vi "TSL_Sample.vi"() -> ()   [LabVIEW 2017]
uses:
  C:/Users/Ssantec_Test/Documents/Instrument_DLL_Sample_Labview_20250826_Ver1.5.0_x64/DLL/InstrumentDLL.dll
  DLL/InstrumentDLL.dll
  <vilib>/Utility/miscctls.llb/LVStringsAndValuesArrayTypeDef_DBL.ctl
  <vilib>/Utility/file.llb/Write To Spreadsheet File (DBL).vi
panel:
  in  "选项卡控件":T1(tab)
  in  "btnUsb_resouce":bool
  out "USB device number":string
  in  "Usb resouce":u16(ring)
  out "SweepSpeed Range":string
  in  "Port number":dbl
  in  "Target":enum32{"rdo550", "rdo570", "rdo770"}(radio)
  in  "btnSplit":bool
  out "GPIB Address":dbl
  out "GPIB Board":dbl
  in  "btnGet_Visa":bool
  in  "Visa String":u16(ring)
  in  "Communication":T2(radio)
  in  "Terminator":enum32{"rdiCr", "rdiLf", "rdiCrLf"}(radio)
  out "Serial":string
  out "Product":string
  out "F/ W Vesion":string
  out "Frequency range":string
  out "Wavelength range":string
  out "APC Limit(dBm)":string
  out "APC Limit(mW)":string
  out "ATT range":string
  in  "Btn_Connect":bool
  in  "Btn_DisConnect":bool
  in  "Address/Device number":string
  out "unit":enum16{"dBm", "mW", ""}(ring)=enum.""
  out "txtshutter":enum16{"Shutter_Open", "Shutter_Close", ""}(ring)=enum.""
  out "status":enum16{"Coh_OFF", "Coh_ON", ""}(ring)=enum.""
  out "mode":enum16{"ACC", "APC", ""}(ring)=enum.""
  out "txtlds":enum16{"LD_OFF", "LD_ON", ""}(ring)=enum.""
  out "LAN Port number":i32
  in  "Get LAN Port":bool
  out "IP Address":string
  in  "Get IP Address":bool
  in  "BtnLD_ON":bool
  in  "BtnLD_OFF":bool
  in  "BtnCoh_ON":bool
  in  "BtnCoh_OFF":bool
  in  "BtnShutter_Open":bool
  in  "BtnShutter_Close":bool
  in  "BtnAPC":bool
  in  "BtnACC":bool
  in  "BtndBm":bool
  in  "BtnmW":bool
  in  "Setting ATT":dbl
  in  "Btn_SetATT":bool
  in  "Setting Power":dbl
  in  "Btn_SetdBm":bool
  in  "Btn_SetmW":bool
  in  "Btn_GetLD":bool
  in  "BtnPower_mode":bool
  in  "BtnCoh_Status":bool
  in  "BtnShutter_Status":bool
  in  "BtnUnit":bool
  out "txtreadatt":dbl
  in  "BtnAtt_value":bool
  out "txtreadpow":dbl
  in  "BtnPower_dBm":bool
  out "txtreadmw":dbl
  in  "BtnPower_mW":bool
  out "txtreadmoni":dbl
  in  "Btnmonitor_dBm":bool
  out "txtradmoni_mw":dbl
  in  "Btnmonitor_mW":bool
  in  "txtsetwave":dbl
  in  "Btn_SetWavelength":bool
  in  "txtsetfreq":dbl
  in  "Btn_SetFrequency":bool
  in  "txtsetft":dbl
  in  "Btn_SetFinetuning":bool
  in  "Btn_Wavelength":bool
  in  "Btn_Frequency":bool
  in  "Btn_Fine":bool
  out "txtwave":dbl
  out "txtfreq":dbl
  out "txtfine":dbl
  out "txtbusy":string
  in  "Btn_Busy":bool
  in  "Wait time(msec)":i32
  in  "Btn_Stangby":bool
  out "txttsl_err":string
  in  "Btn_error":bool
  out "Start mode":enum16{"Normal", "WaitingforTrigger", ""}(ring)=enum.""
  out "Trigger output":enum16{"None", "Stop", "Start", "Step", ""}(ring)=enum.""
  out "Trigger input":enum16{"Disable", "Enable", ""}(ring)=enum.""
  out "Sweep Mode":T3(ring)=enum.""
  out "txtg_sweep_su":T4(ring)=enum."Returning"
  out "Trigger Source":enum16{"Wavelength", "Time", ""}(ring)=enum.""
  in  "Speed(570)":u16(ring) caption="Speed(nm/sec)" items=["1"=1, "2"=2, "5"=5, "10"=10, "20"=20, "50"=50, "100"=100, "200"=200]
  in  "Speed":u16(ring)
  in  "Get speed table":bool
  in  "cmbTrigger_Source":u16(ring) caption="Trigger Source(570)" items=["Wavelength", "Time", ""]
  in  "txtstart":dbl caption="Start wavelength"
  in  "Btn_SetWavelength_Parameters":bool
  in  "txtstop":dbl caption="Stop wavelength"
  in  "txtstep":dbl=0.1 caption="Trigger/wave step"
  in  "txtspeed(550)":dbl caption="Speed(nm/sec)"
  in  "Btn_Other":bool
  in  "txtdelay":dbl caption="Delay time(sec)"
  in  "txtcycle":i32=1 caption="cycle"
  in  "cmbsm":u16(ring) caption="Sweep Mode" items=["Step one way", "Continuous one way", "Step round trip", "Continuous round trip"]
  in  "cmbst_mod":u16(ring) caption="Trigger input" items=["Disable", "Enable"]
  in  "cmbtout":u16(ring) caption="Trigger output" items=["None", "Stop", "Start", "Step"]
  in  "cmbtin":u16(ring) caption="Start mode" items=["Normal", "Waiting for Trigger"]
  out "Start wavelength":dbl
  out "Stop wavelength":dbl
  out "Wavelength step":dbl
  out "Trigger step":dbl
  out "Speed(nm/sec)":dbl
  out "Delay time(sec)":dbl
  out "cycle":i32
  in  "BtnGet_setting":bool
  in  "Status":u16(ring) items=["Standby", "Running", "Pauseing", "WaitingforTrigger", "Returning"]
  in  "Wait time(msec)":i32
  in  "Btn_Waiting":bool
  in  "Btn_Status":bool
  in  "Btn_Minstep":bool
  in  "txtspeed":dbl
  out "txtcurrentc":i32
  in  "Btn_Current":bool
  in  "Btn_Start":bool
  in  "Btn_Stop":bool
  in  "Btn_SoftwareTrigger":bool
  in  "Btn_Pause":bool
  in  "Btn_ReStart":bool
  in  "Btn_GetLogg":bool
  out "TSL":refnum<k24>
  # "0. Connect Tool"
  # "1. Connect"
  # "Information"
  # "Power Control"
  # "Power status"
  # "Wavelength Control"
  # "Wavelength Status"
  # "Common Function"
  # "Sweep Setting"
  # "Other"
  # "Wavelength parameters"
  # "Other parameters"
  # "Sweep Speed(nm/s)"
  # "Sweep setting status"
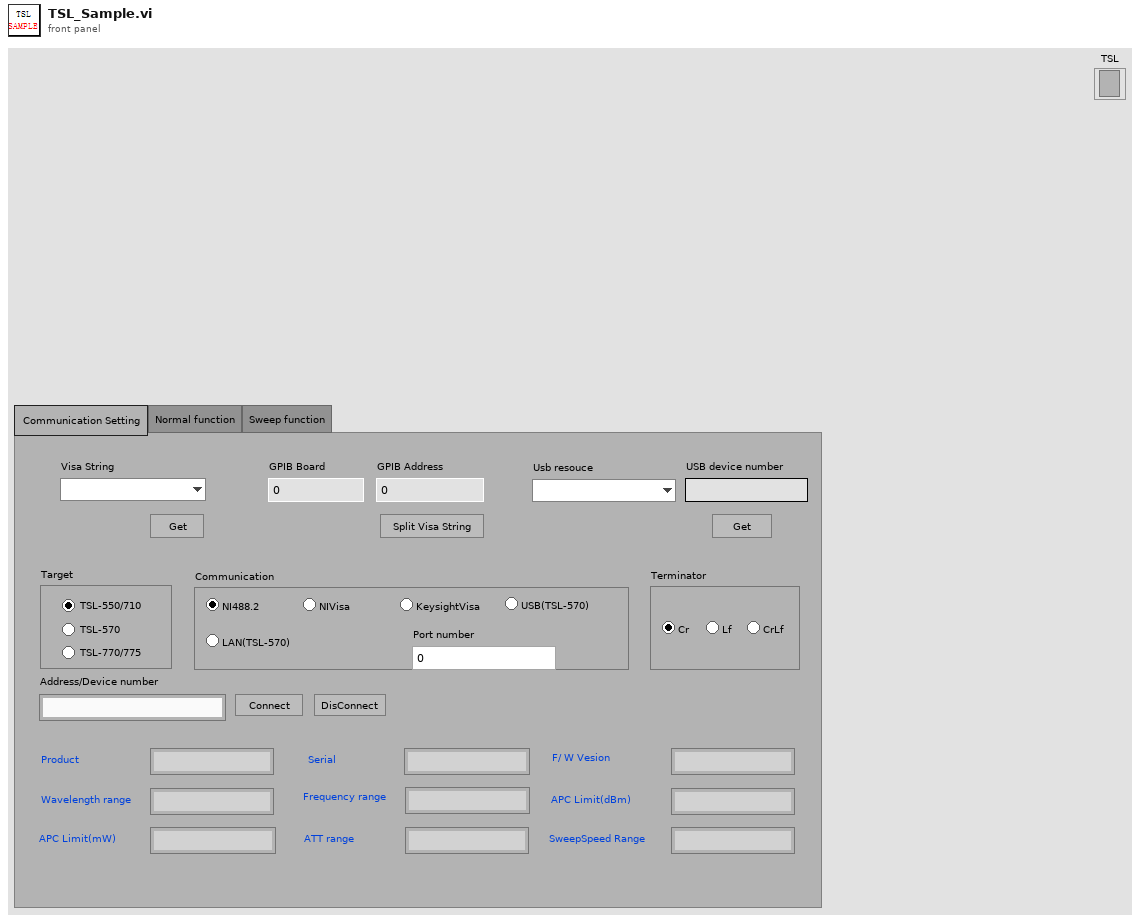
[diagram p1: front panel]
types:
  T1 = enum32{"Communication Setting ", "Normal function", "Sweep function"}
  T2 = enum32{"rdiNI488", "rdiNIvisa", "rdikysightvisa", "rdiUSB", "rdiLAN"}
  T3 = enum16{"Step_Oneway", "Continuous_Oneway", "Step_Twoway", "Continuous_Twoway", ""}
  T4 = enum16{"Standby", "Running", "Pausing", "WaitingforTrigger", "Returning"}
  T5 = enum16{"Standby", "Running", "Pausing", "WaitingforTrigger", "Returning", ""}
  T6 = enum8{"Enabled", "Disabled", "Disabled and Grayed Out"}
  T7 = typedef "LVStringsAndValuesArrayTypeDef_DBL.ctl" = cluster{"String":string, "Value":dbl}[]
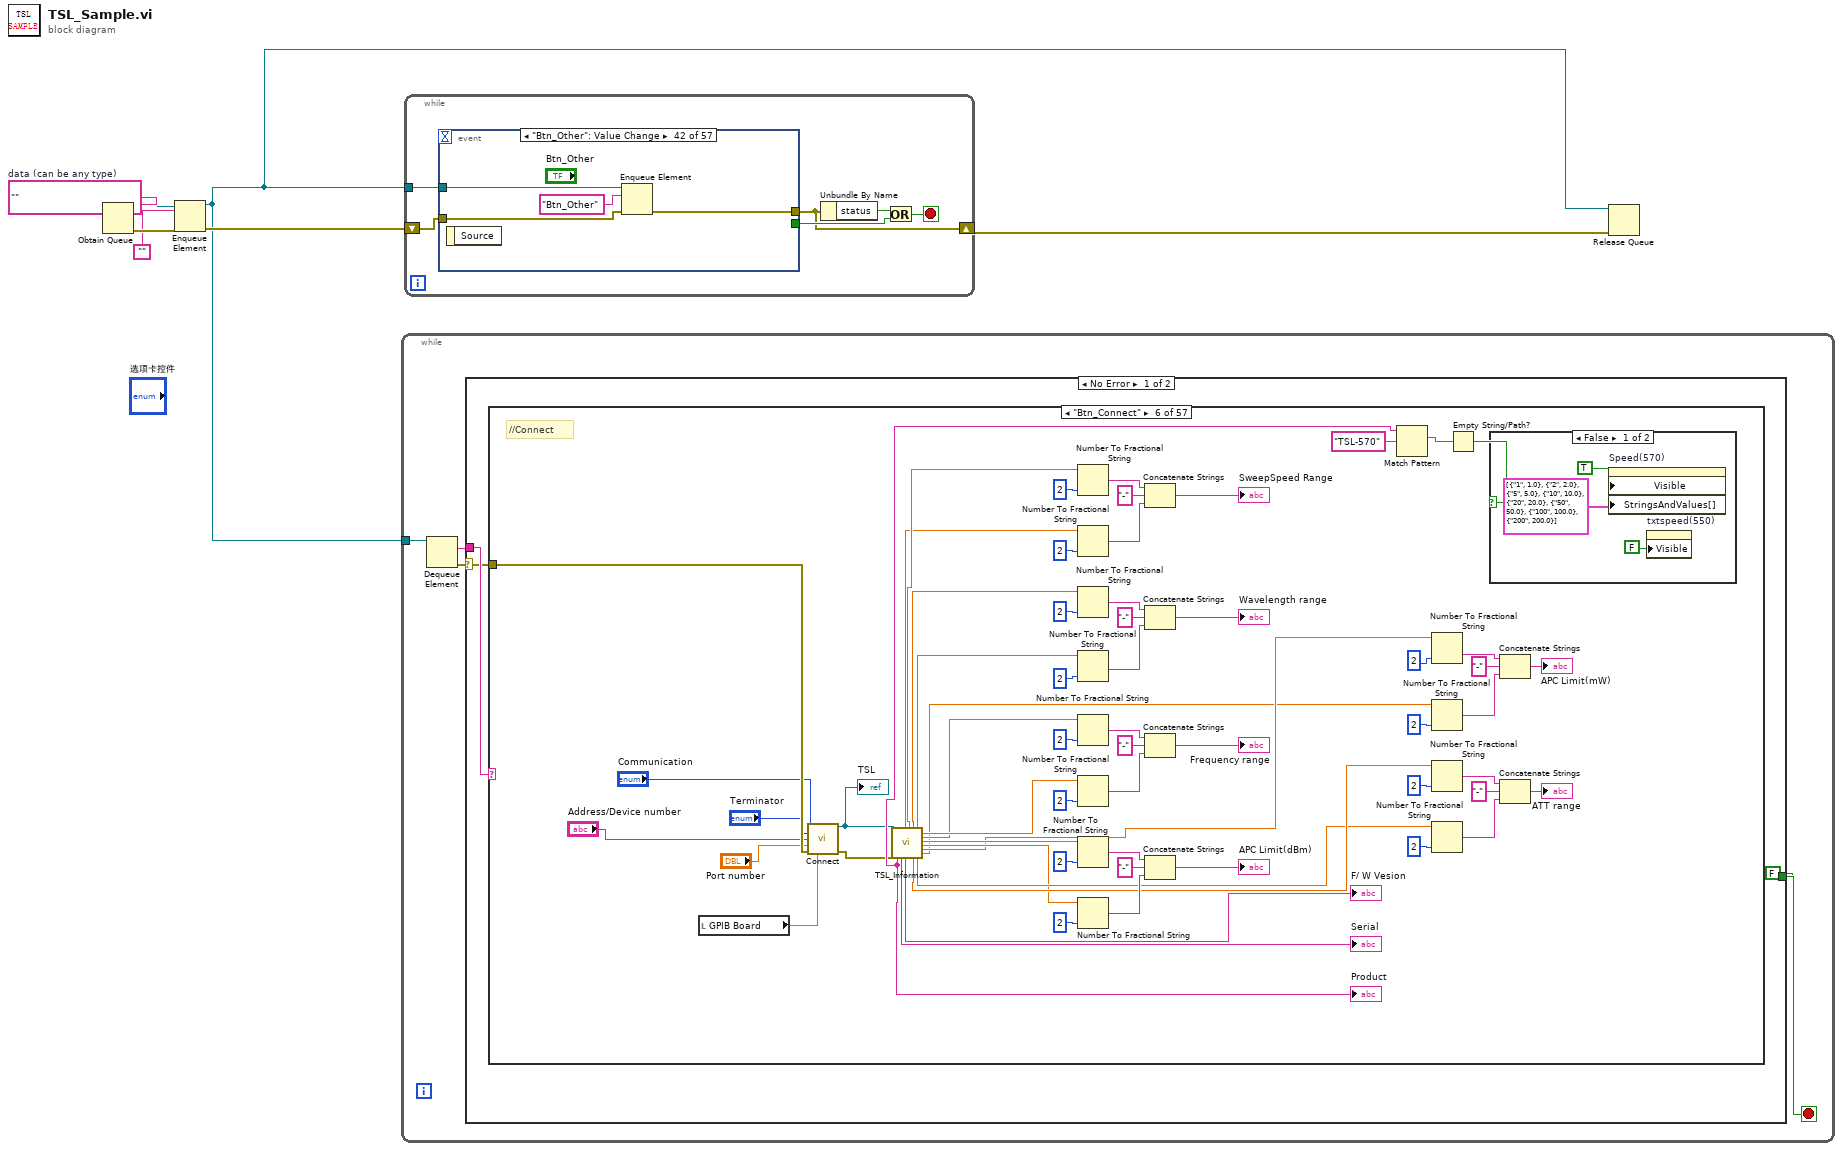
[diagram p0: block diagram]
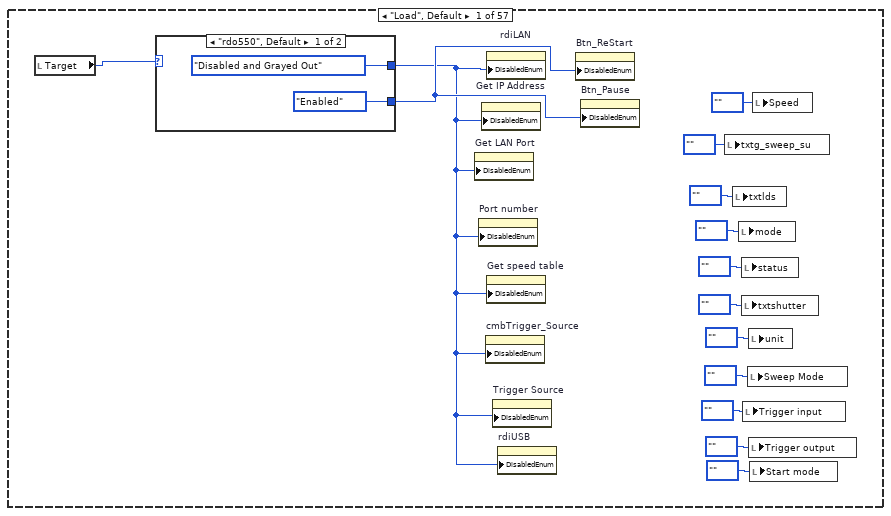
[diagram p2: hidden frame]
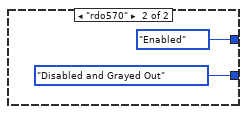
[diagram p3: hidden frame]
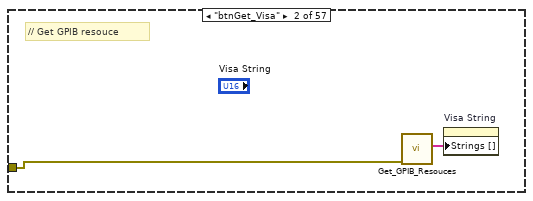
[diagram p4: hidden frame]
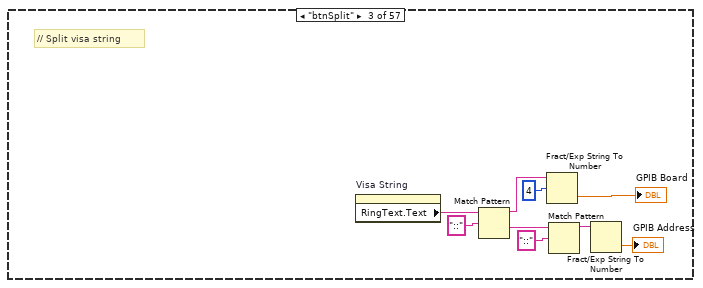
[diagram p5: hidden frame]
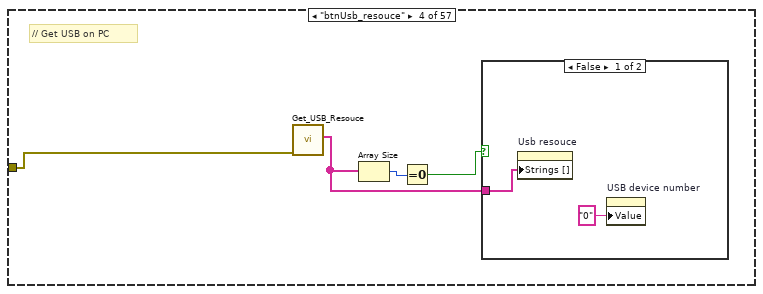
[diagram p6: hidden frame]
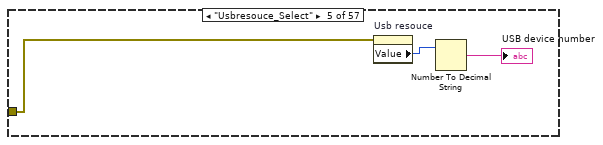
[diagram p8: hidden frame]
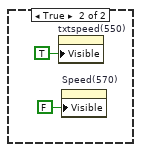
[diagram p9: hidden frame]
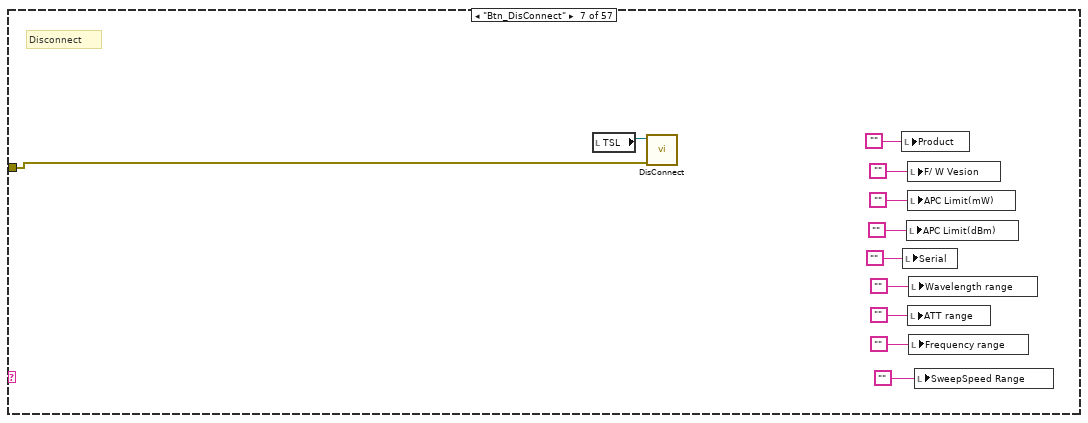
[diagram p10: hidden frame]
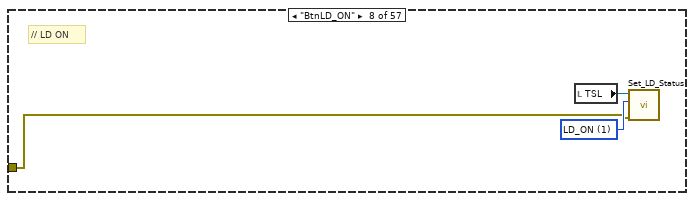
[diagram p11: hidden frame]
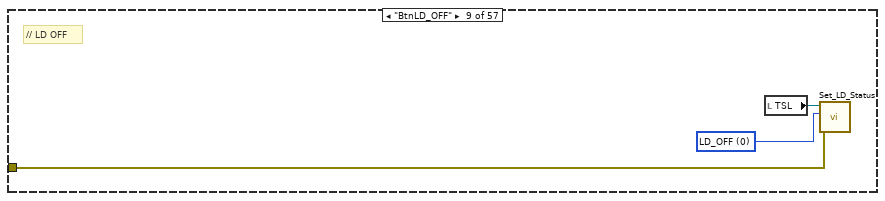
[diagram p12: hidden frame]
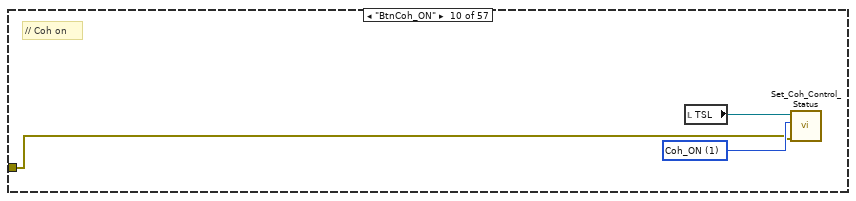
[diagram p13: hidden frame]
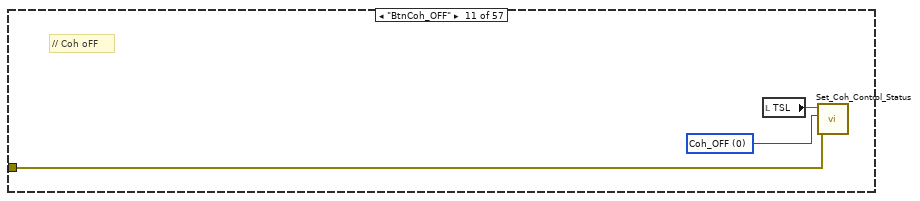
[diagram p14: hidden frame]
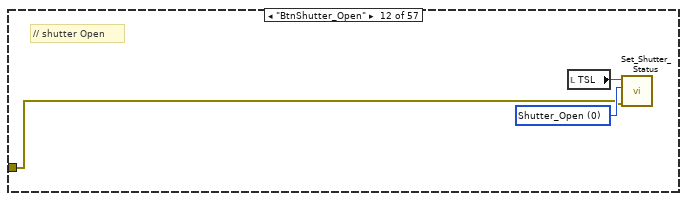
[diagram p15: hidden frame]
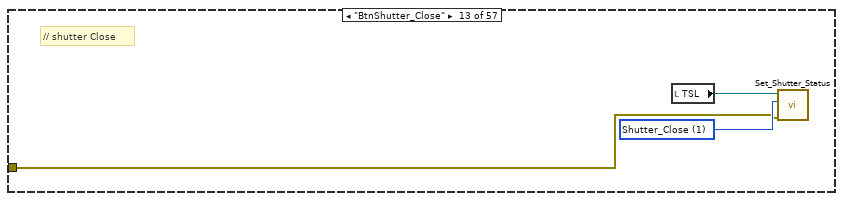
[diagram p16: hidden frame]
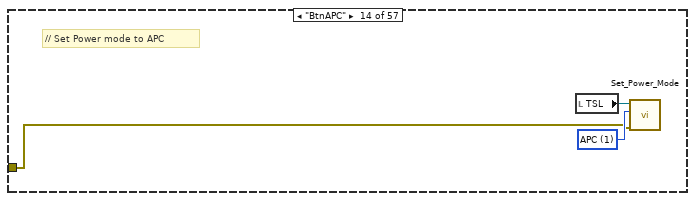
[diagram p17: hidden frame]
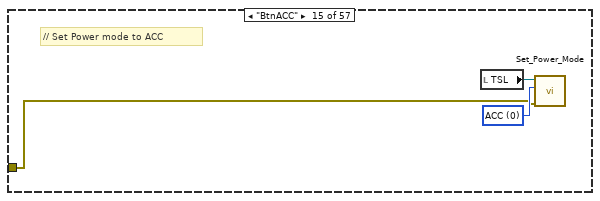
[diagram p18: hidden frame]
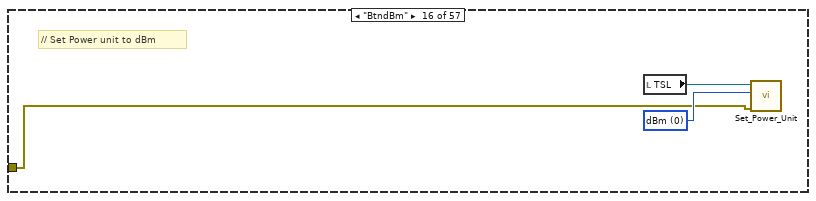
[diagram p19: hidden frame]
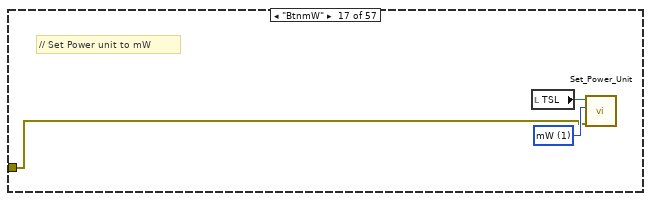
[diagram p20: hidden frame]
diagram:
  w4 = ""  # data (can be any type)
  n1 = Obtain Queue(element data type=w4) -> (queue out=w3:refnum<queue>, error out=w7:errorcluster)  [unwired: 4 in, 1 out]
  n2 = Enqueue Element(queue=w3, element="", error in (no error)=w7) -> (queue out=w1:refnum<queue>, error out=w6:errorcluster)  [unwired: 1 in, 1 out]
  n3 = while {
    tunnel: w1 -> [w11]
    stop <- w8 stop-if-true
    n4 = Dequeue Element(queue=w11) -> (element=w9:string, error out=w10:errorcluster)  [unwired: 2 in, 2 out]
    n5 = case shown="No Error" w10 {
      selector: w10 -> [w12 _]
      tunnel: w9 -> [w14 _]
      tunnel: [FALSE TRUE] -> w8
      frame No Error {
        n6 = case shown="\"Btn_Connect\"" w14 {
          tunnel: w12 -> [_ w33 _ w44 w52 w59 w120 w131 w134 w137 w140 w143 w146 w149 w152 w155 w158 w161 w164 w168 w170 w173 w176 w179 w182 w185 w188 w193 w207 _ w238 w242 w244 w248 w251 w254 w256 w259 w262 w265 w268 w271 w280 w307 w346 w361 w364 w367 w370 w378 w380 w382 w384 w388 w390 w393 _]
          frame "Load", Default {
            n7 = local read "Target"() -> (w27:enum32{"rdo550", "rdo570", "rdo770"})
            n8 = case shown="\"rdo550\", Default" w27 {
              tunnel: [T6."Disabled and Grayed Out" ("禁用") T6."Enabled" ("禁用")] -> w26
              tunnel: [T6."Enabled" ("禁用") T6."Disabled and Grayed Out" ("禁用")] -> w28
              frame "rdo550", Default {
              }
              frame "rdo570" {
              }
            }
            n9 = property on="Get LAN Port" class="Bool"("DisabledEnum"=w26) -> ()  [unwired: 2 in, 2 out]
            n10 = property on="Port number" class="DigNum (strict)"("DisabledEnum"=w26) -> ()  [unwired: 2 in, 2 out]
            n11 = property on="Get IP Address" class="Bool"("DisabledEnum"=w26) -> ()  [unwired: 2 in, 2 out]
            n12 = property on="cmbTrigger_Source" class="Ring (strict)"("DisabledEnum"=w26) -> ()  [unwired: 2 in, 2 out]
            n13 = property on="rdiLAN" class="Bool (strict)"("DisabledEnum"=w26) -> ()  [unwired: 2 in, 2 out]
            n14 = property on="Get speed table" class="Bool"("DisabledEnum"=w26) -> ()  [unwired: 2 in, 2 out]
            n15 = property on="Trigger Source" class="Enum (strict)"("DisabledEnum"=w26) -> ()  [unwired: 2 in, 2 out]
            n16 = property on="rdiUSB" class="Bool (strict)"("DisabledEnum"=w26) -> ()  [unwired: 2 in, 2 out]
            n17 = property on="Btn_ReStart" class="Bool"("DisabledEnum"=w28) -> ()  [unwired: 2 in, 2 out]
            n18 = property on="Btn_Pause" class="Bool"("DisabledEnum"=w28) -> ()  [unwired: 2 in, 2 out]
            n19 = local write "txtg_sweep_su"(T5."" ("txtg_sweep_su")) -> ()
            n20 = local write "txtlds"(enum16{"LD_OFF", "LD_ON", ""}."" ("txtlds")) -> ()
            n21 = local write "mode"(enum16{"ACC", "APC", ""}."" ("mode")) -> ()
            n22 = local write "status"(enum16{"Coh_OFF", "Coh_ON", ""}."" ("status")) -> ()
            n23 = local write "txtshutter"(enum16{"Shutter_Open", "Shutter_Close", ""}."" ("txtshutter")) -> ()
            n24 = local write "Trigger input"(enum16{"Disable", "Enable", ""}."" ("Trigger input")) -> ()
            n25 = local write "Sweep Mode"(T3."" ("Sweep Mode")) -> ()
            n26 = local write "unit"(enum16{"dBm", "mW", ""}."" ("unit")) -> ()
            n27 = local write "Trigger output"(enum16{"None", "Stop", "Start", "Step", ""}."" ("Trigger output")) -> ()
            n28 = local write "Start mode"(enum16{"Normal", "WaitingforTrigger", ""}."" ("Start mode")) -> ()
            n29 = local write "Speed"(enum16{""}."" ("Speed")) -> ()
          }
          frame "btnGet_Visa" {
            # "// Get GPIB resouce"
            n30 = call "Get_GPIB_Resouces.vi"("error in (no error)"=w33) -> ("Get_GPIB_Resources"=w34:string[])  [unwired: 8 in, 2 out]
            n31 = property on="Visa String" class="Ring (strict)"("Strings []"=w34) -> ()  [unwired: 2 in, 2 out]
          }
          frame "btnSplit" {
            # "// Split visa string"
            n32 = property on="Visa String" class="Ring (strict)"() -> ("RingText.Text"=w43:string)  [unwired: 2 in, 2 out]
            n33 = Match Pattern(string=w43, regular expression="::") -> (before substring=w39:string, after substring=w40:string)  [unwired: 1 in, 2 out]
            n34 = Fract/Exp String To Number(string=w39, offset=4 ("偏移量")) -> (number=→"GPIB Board":dbl)  [unwired: 2 in, 1 out]
            n35 = Match Pattern(string=w40, regular expression="::") -> (before substring=w36:string)  [unwired: 1 in, 3 out]
            n36 = Fract/Exp String To Number(string=w36) -> (number=→"GPIB Address":dbl)  [unwired: 3 in, 1 out]
          }
          frame "btnUsb_resouce" {
            # "// Get USB on PC"
            n37 = call "Get_USB_Resouce.vi"("error in (no error)"=w44) -> ("Get_USB_Resouce"=w45:string[])  [unwired: 8 in, 2 out]
            n38 = Array Size(array=w45) -> (size(s)=w47:i32)
            n39 = Equal To 0?(x=w47) -> (x = 0?=w46:bool)
            n40 = case shown="False" w46 {
              tunnel: w45 -> [w49 _]
              frame False {
                n41 = property on="Usb resouce" class="Ring (strict)"("Strings []"=w49) -> ()  [unwired: 2 in, 2 out]
                n42 = property on="USB device number" class="Str"("Value"="0" ("USB device number")) -> ()  [unwired: 2 in, 2 out]
              }
              frame True {
              }
            }
          }
          frame "Usbresouce_Select" {
            n43 = property on="Usb resouce" class="Ring (strict)"(error in=w52) -> ("Value"=w51:u16)  [unwired: 1 in, 2 out]
            n44 = Number To Decimal String(number=w51) -> (decimal integer string=→"USB device number":string)  [unwired: 1 in]
          }
          frame "Btn_Connect" {
            # "//Connect"
            n45 = local read "GPIB Board"() -> (w53:dbl)
            n46 = call "Connect.vi"("Communication"="Communication", "Terminator"="Terminator", "Address/Device number"="Address/Device number", "Port"="Port number", "error in (no error)"=w59, "GPIBBoard"=w53) -> ("Reference out"=w60:refnum<k24>, "error out"=w58:errorcluster)  [unwired: 8 in]
            "TSL" <- w60
            n47 = call "TSL_Information.vi"(".NET Reference in"=w60, "error in (no error)"=w58) -> ("ProductName"=w61:string, "SerialNumber"=→"Serial":string, "MaximumSpeed"=w70:dbl, "FWversion"=→"F/ W Vesion":string, "MinimumSpeed"=w71:dbl, "MinimunWavelength"=w69:dbl, "MinimumATTValue"=w73:dbl, "MaximumWavelength"=w68:dbl, "MaximumATTValue"=w72:dbl, "MaximumFrequency"=w67:dbl, "MinimunFrequency"=w66:dbl, "MinimumAPCPower_dBm"=w65:dbl, "MaximumAPCPower_dBm"=w64:dbl, "MinimumAPCPower_mW"=w63:dbl, "MaximumAPCPower_mW"=w62:dbl)  [unwired: 9 in, 2 out]
            "Product" <- w61
            n48 = Number To Fractional String(number=w71, precision (6)=i16 2 ("精度(6)")) -> (F-format string=w83:string)  [unwired: 2 in]
            n49 = Number To Fractional String(number=w70, precision (6)=i16 2 ("精度(6)")) -> (F-format string=w82:string)  [unwired: 2 in]
            n50 = Number To Fractional String(number=w69, precision (6)=i16 2 ("精度(6)")) -> (F-format string=w109:string)  [unwired: 2 in]
            n51 = Number To Fractional String(number=w68, precision (6)=i16 2 ("精度(6)")) -> (F-format string=w110:string)  [unwired: 2 in]
            n52 = Number To Fractional String(number=w66, precision (6)=i16 2 ("精度(6)")) -> (F-format string=w114:string)  [unwired: 2 in]
            n53 = Number To Fractional String(number=w67, precision (6)=i16 2 ("精度(6)")) -> (F-format string=w113:string)  [unwired: 2 in]
            n54 = Number To Fractional String(number=w65, precision (6)=i16 2 ("精度(6)")) -> (F-format string=w105:string)  [unwired: 2 in]
            n55 = Number To Fractional String(number=w64, precision (6)=i16 2 ("精度(6)")) -> (F-format string=w104:string)  [unwired: 2 in]
            n56 = Concatenate Strings(w83, "-" ("字符串"), w82) -> (→"SweepSpeed Range":string)
            n57 = Concatenate Strings(w109, "-" ("字符串"), w110) -> (→"Wavelength range":string)
            n58 = Concatenate Strings(w114, "-" ("字符串"), w113) -> (→"Frequency range":string)
            n59 = Concatenate Strings(w105, "-" ("字符串"), w104) -> (→"APC Limit(dBm)":string)
            n60 = Match Pattern(string=w61, regular expression="TSL-570" ("正则表达式")) -> (match substring=w77:string)  [unwired: 1 in, 3 out]
            n61 = Number To Fractional String(number=w63, precision (6)=i16 2 ("精度(6)")) -> (F-format string=w102:string)  [unwired: 2 in]
            n62 = Number To Fractional String(number=w62, precision (6)=i16 2 ("精度(6)")) -> (F-format string=w101:string)  [unwired: 2 in]
            n63 = Number To Fractional String(number=w73, precision (6)=i16 2 ("精度(6)")) -> (F-format string=w107:string)  [unwired: 2 in]
            n64 = Number To Fractional String(number=w72, precision (6)=i16 2 ("精度(6)")) -> (F-format string=w106:string)  [unwired: 2 in]
            n65 = Empty String/Path?(string/path=w77) -> (empty?=w76:bool)
            n66 = case shown="False" w76 {
              frame False {
                n67 = property on="Speed(570)" class="Ring (strict)"("Visible"=TRUE ("可见"), "StringsAndValues[]"=T7 [{"String"="1", "Value"=1.0}, {"String"="2", "Value"=2.0}, {"String"="5", "Value"=5.0}, {"String"="10", "Value"=10.0}, {"String"="20", "Value"=20.0}, {"String"="50", "Value"=50.0}, {"String"="100", "Value"=100.0}, {"String"="200", "Value"=200.0}] ("Strings And Values []")) -> ()  [unwired: 2 in, 2 out]
                n68 = property on="txtspeed(550)" class="DigNum (strict)"("Visible"=FALSE ("可见")) -> ()  [unwired: 2 in, 2 out]
              }
              frame True {
                n69 = property on="txtspeed(550)" class="DigNum (strict)"("Visible"=TRUE ("可见")) -> ()  [unwired: 2 in, 2 out]
                n70 = property on="Speed(570)" class="Ring (strict)"("Visible"=FALSE ("可见")) -> ()  [unwired: 2 in, 2 out]
              }
            }
            n71 = Concatenate Strings(w102, "-" ("字符串"), w101) -> (→"APC Limit(mW)":string)
            n72 = Concatenate Strings(w107, "-" ("字符串"), w106) -> (→"ATT range":string)
          }
          frame "Btn_DisConnect" {
            # "Disconnect"
            n73 = local read "TSL"() -> (w122:refnum<k24>)
            n74 = call "DisConnect.vi"("error in (no error)"=w120, ".NET Reference in"=w122) -> ()  [unwired: 4 in, 2 out]
            n75 = local write "Product"("") -> ()
            n76 = local write "Serial"("") -> ()
            n77 = local write "APC Limit(dBm)"("") -> ()
            n78 = local write "F/ W Vesion"("") -> ()
            n79 = local write "APC Limit(mW)"("") -> ()
            n80 = local write "ATT range"("") -> ()
            n81 = local write "Wavelength range"("") -> ()
            n82 = local write "Frequency range"("") -> ()
            n83 = local write "SweepSpeed Range"("") -> ()
          }
          frame "BtnLD_ON" {
            w133 = 1 items=["LD_OFF", "LD_ON"] ("status 2")
            # "// LD ON"
            n84 = local read "TSL"() -> (w132:refnum<k24>)
            n85 = call "Set_LD_Status.vi"("error in (no error)"=w131, "status"=w133, ".NET Reference in"=w132) -> ()  [unwired: 7 in, 2 out]
          }
          frame "BtnLD_OFF" {
            w135 = 0 items=["LD_OFF", "LD_ON"] ("status 2")
            # "// LD OFF"
            n86 = local read "TSL"() -> (w136:refnum<k24>)
            n87 = call "Set_LD_Status.vi"("error in (no error)"=w134, "status"=w135, ".NET Reference in"=w136) -> ()  [unwired: 7 in, 2 out]
          }
          frame "BtnCoh_ON" {
            w138 = 1 items=["Coh_OFF", "Coh_ON"] ("status 2")
            # "// Coh on"
            n88 = local read "TSL"() -> (w139:refnum<k24>)
            n89 = call "Set_Coh_Control_Status.vi"(".NET Reference in"=w139, "status"=w138, "error in (no error)"=w137) -> ()  [unwired: 6 in, 2 out]
          }
          frame "BtnCoh_OFF" {
            w141 = 0 items=["Coh_OFF", "Coh_ON"] ("status 2")
            # "// Coh oFF"
            n90 = local read "TSL"() -> (w142:refnum<k24>)
            n91 = call "Set_Coh_Control_Status.vi"(".NET Reference in"=w142, "status"=w141, "error in (no error)"=w140) -> ()  [unwired: 6 in, 2 out]
          }
          frame "BtnShutter_Open" {
            w144 = 0 items=["Shutter_Open", "Shutter_Close"] ("status 2")
            # "// shutter Open"
            n92 = local read "TSL"() -> (w145:refnum<k24>)
            n93 = call "Set_Shutter_Status.vi"(".NET Reference in"=w145, "status"=w144, "error in (no error)"=w143) -> ()  [unwired: 6 in, 2 out]
          }
          frame "BtnShutter_Close" {
            w147 = 1 items=["Shutter_Open", "Shutter_Close"] ("status 2")
            # "// shutter Close"
            n94 = local read "TSL"() -> (w148:refnum<k24>)
            n95 = call "Set_Shutter_Status.vi"(".NET Reference in"=w148, "status"=w147, "error in (no error)"=w146) -> ()  [unwired: 6 in, 2 out]
          }
          frame "BtnAPC" {
            w150 = 1 items=["ACC", "APC"] ("mode")
            # "// Set Power mode to APC"
            n96 = local read "TSL"() -> (w151:refnum<k24>)
            n97 = call "Set_Power_Mode.vi"(".NET Reference in"=w151, "mode"=w150, "error in (no error)"=w149) -> ()  [unwired: 6 in, 2 out]
          }
          frame "BtnACC" {
            w153 = 0 items=["ACC", "APC"] ("mode")
            # "// Set Power mode to ACC"
            n98 = local read "TSL"() -> (w154:refnum<k24>)
            n99 = call "Set_Power_Mode.vi"(".NET Reference in"=w154, "mode"=w153, "error in (no error)"=w152) -> ()  [unwired: 6 in, 2 out]
          }
          frame "BtndBm" {
            w156 = 0 items=["dBm", "mW"] ("unit")
            # "// Set Power unit to dBm"
            n100 = local read "TSL"() -> (w157:refnum<k24>)
            n101 = call "Set_Power_Unit.vi"(".NET Reference in"=w157, "unit"=w156, "error in (no error)"=w155) -> ()  [unwired: 6 in, 2 out]
          }
          frame "BtnmW" {
            w159 = 1 items=["dBm", "mW"] ("unit")
            # "// Set Power unit to mW"
            n102 = local read "TSL"() -> (w160:refnum<k24>)
            n103 = call "Set_Power_Unit.vi"(".NET Reference in"=w160, "unit"=w159, "error in (no error)"=w158) -> ()  [unwired: 6 in, 2 out]
          }
          frame "Btn_SetATT" {
            # "// SetATT"
            n104 = local read "TSL"() -> (w163:refnum<k24>)
            n105 = call "Set_Att_Value.vi"(".NET Reference in"=w163, "Setting ATT"="Setting ATT", "error in (no error)"=w161) -> ()  [unwired: 5 in, 2 out]
          }
          frame "Btn_SetdBm" {
            # "// Set Power dBm"
            n106 = local read "TSL"() -> (w166:refnum<k24>)
            n107 = call "Set_APC_Power_dBm.vi"(".NET Reference in"=w166, "Setting Power"="Setting Power", "error in (no error)"=w164) -> ()  [unwired: 6 in, 2 out]
          }
          frame "Btn_SetmW" {
            # "// Set Power mW"
            n108 = local read "Setting Power"() -> (w167:dbl)
            n109 = local read "TSL"() -> (w169:refnum<k24>)
            n110 = call "Set_APC_Power_mW.vi"(".NET Reference in"=w169, "Setting Power"=w167, "error in (no error)"=w168) -> ()  [unwired: 6 in, 2 out]
          }
          frame "Btn_SetWavelength" {
            # "// set Wavelength"
            n111 = local read "TSL"() -> (w172:refnum<k24>)
            n112 = call "Set_Wavelength.vi"("error in (no error)"=w170, "txtsetwave"="txtsetwave", ".NET Reference in"=w172) -> ()  [unwired: 3 in, 2 out]
          }
          frame "Btn_SetFrequency" {
            # "// set Frequency"
            n113 = local read "TSL"() -> (w175:refnum<k24>)
            n114 = call "Set_Frequency.vi"("error in (no error)"=w173, "txtsetfreq"="txtsetfreq", ".NET Reference in"=w175) -> ()  [unwired: 7 in, 2 out]
          }
          frame "Btn_SetFinetuning" {
            # "// Set Finetuning"
            n115 = local read "TSL"() -> (w178:refnum<k24>)
            n116 = call "Set_Finetuning.vi"("error in (no error)"=w176, "txtsetft"="txtsetft", ".NET Reference in"=w178) -> ()  [unwired: 7 in, 2 out]
          }
          frame "Btn_Wavelength" {
            # "// Get Setting Wavelength Value"
            n117 = local read "TSL"() -> (w180:refnum<k24>)
            n118 = call "Get_Wavelength.vi"("error in (no error)"=w179, ".NET Reference in"=w180) -> ("wav"=→"txtwave":dbl)  [unwired: 7 in, 2 out]
          }
          frame "Btn_Frequency" {
            # "// Get Setting Frequency"
            n119 = local read "TSL"() -> (w183:refnum<k24>)
            n120 = call "Get_Frequency.vi"("error in (no error)"=w182, ".NET Reference in"=w183) -> ("freq"=→"txtfreq":dbl)  [unwired: 7 in, 2 out]
          }
          frame "Btn_Fine" {
            # "// Get Fine tuning value"
            n121 = local read "TSL"() -> (w186:refnum<k24>)
            n122 = call "Get_Finetuning.vi"("error in (no error)"=w185, ".NET Reference in"=w186) -> ("ftval"=→"txtfine":dbl)  [unwired: 7 in, 2 out]
          }
          frame "Btn_Busy" {
            # "// Get Busy status"
            n123 = local read "TSL"() -> (w190:refnum<k24>)
            n124 = call "Get_Busy_Status.vi"("error in (no error)"=w188, ".NET Reference in"=w190) -> ("busyflag"=w189:bool)  [unwired: 7 in, 2 out]
            n125 = case shown="True" w189 {
              frame False {
                n126 = local write "txtbusy"("Standby") -> ()
              }
              frame True {
                "txtbusy" <- "Busy"
              }
            }
          }
          frame "Btn_Stangby" {
            # "// Waiting for standby until wait time"
            n127 = flat-sequence {
              tunnel: [w201] -> w195
              tunnel: w193 -> [w203]
              tunnel: [w205] -> w194
              frame #0 {
                n128 = Tick Count (ms)() -> (millisecond timer value=w201:u32)
              }
              frame #1 {
                n129 = local read "TSL"() -> (w204:refnum<k24>)
                n130 = call "TSL_Busy_Check.vi"("error in (no error)"=w203, "Wait time(msec)"="Wait time(msec)", ".NET Reference in"=w204) -> ()  [unwired: 7 in, 2 out]
              }
              frame #2 {
                n131 = Tick Count (ms)() -> (millisecond timer value=w205:u32)
              }
            }
            n132 = Subtract(x=w194, y=w195) -> (x-y=w196:u32)
            n133 = Number To Decimal String(number=w196) -> (decimal integer string=w199:string)  [unwired: 1 in]
            n134 = Concatenate Strings("Busy time :", w199, "ms") -> (w197:string)
            n135 = One Button Dialog(message=w197) -> ()  [unwired: 1 in, 1 out]
          }
          frame "Get speed table" {
            n136 = local read "TSL"() -> (w206:refnum<k24>)
            n137 = local read "Target"() -> (w208:enum32{"rdo550", "rdo570", "rdo770"})
            n138 = case shown="\"rdo770\"" w208 {
              tunnel: w207 -> [_ w212 w222]
              tunnel: w206 -> [_ w209 w219]
              frame "rdo550", Default {
              }
              frame "rdo570" {
                n139 = call "Get_Sweep_Speed_table.vi"("error in (no error)"=w212, ".NET Reference in"=w209) -> ("error out"=w211:errorcluster, "Get_Sweep_Speed_table"=w214:dbl[])  [unwired: 7 in, 1 out]
                n140 = for {
                  tunnel: w214 -> [w218] mode=indexing
                  shift-right: [w215] -> w210
                  shift-left: string[] [] ("添加的数组") -> [w216]
                  n141 = Number To Decimal String(number=w218) -> (decimal integer string=w217:string)  [unwired: 1 in]
                  n142 = Build Array (concatenate)(w216, w217) -> (w215:string[])
                }
                n143 = property on="Speed" class="Ring (strict)"(error in=w211, "Strings []"=w210) -> ()  [unwired: 1 in, 2 out]
              }
              frame "rdo770" {
                n144 = call "Get_Sweep_Speed_table.vi"("error in (no error)"=w222, ".NET Reference in"=w219) -> ("error out"=w221:errorcluster, "Get_Sweep_Speed_table"=w224:dbl[])  [unwired: 7 in, 1 out]
                n145 = for {
                  tunnel: w224 -> [w228] mode=indexing
                  shift-right: [w225] -> w220
                  shift-left: string[] [] ("添加的数组") -> [w226]
                  n146 = Number To Decimal String(number=w228) -> (decimal integer string=w227:string)  [unwired: 1 in]
                  n147 = Build Array (concatenate)(w226, w227) -> (w225:string[])
                }
                n148 = property on="Speed" class="Ring (strict)"(error in=w221, "Strings []"=w220) -> ()  [unwired: 1 in, 2 out]
              }
            }
          }
          frame "Target" {
            n149 = case shown="\"rdo570\"" "Target" {
              tunnel: [T6."Enabled" ("禁用") T6."Disabled and Grayed Out" ("禁用") w236] -> w230
              tunnel: [w232 w234 T6."Disabled and Grayed Out" ("禁用")] -> w229
              frame "rdo770" {
                w232 = T6."Disabled and Grayed Out" ("禁用")
                n150 = property on="Btn_SetATT" class="Bool"("DisabledEnum"=w232) -> ()  [unwired: 2 in, 2 out]
                n151 = property on="BtnAtt_value" class="Bool"("DisabledEnum"=w232) -> ()  [unwired: 2 in, 2 out]
              }
              frame "rdo550", Default {
                w234 = T6."Enabled" ("禁用")
                n152 = property on="Btn_SetATT" class="Bool"("DisabledEnum"=w234) -> ()  [unwired: 2 in, 2 out]
                n153 = property on="BtnAtt_value" class="Bool"("DisabledEnum"=w234) -> ()  [unwired: 2 in, 2 out]
              }
              frame "rdo570" {
                w236 = T6."Enabled" ("禁用")
                n154 = property on="Btn_SetATT" class="Bool"("DisabledEnum"=w236) -> ()  [unwired: 2 in, 2 out]
                n155 = property on="BtnAtt_value" class="Bool"("DisabledEnum"=w236) -> ()  [unwired: 2 in, 2 out]
              }
            }
            n156 = property on="Get LAN Port" class="Bool"("DisabledEnum"=w230) -> ()  [unwired: 2 in, 2 out]
            n157 = property on="Port number" class="DigNum (strict)"("DisabledEnum"=w230) -> ()  [unwired: 2 in, 2 out]
            n158 = property on="Get IP Address" class="Bool"("DisabledEnum"=w230) -> ()  [unwired: 2 in, 2 out]
            n159 = property on="cmbTrigger_Source" class="Ring (strict)"("DisabledEnum"=w230) -> ()  [unwired: 2 in, 2 out]
            n160 = property on="rdiLAN" class="Bool (strict)"("DisabledEnum"=w230) -> ()  [unwired: 2 in, 2 out]
            n161 = property on="Get speed table" class="Bool"("DisabledEnum"=w230) -> ()  [unwired: 2 in, 2 out]
            n162 = property on="Trigger Source" class="Enum (strict)"("DisabledEnum"=w230) -> ()  [unwired: 2 in, 2 out]
            n163 = property on="rdiUSB" class="Bool (strict)"("DisabledEnum"=w230) -> ()  [unwired: 2 in, 2 out]
            n164 = property on="Btn_ReStart" class="Bool"("DisabledEnum"=w229) -> ()  [unwired: 2 in, 2 out]
            n165 = property on="Btn_Pause" class="Bool"("DisabledEnum"=w229) -> ()  [unwired: 2 in, 2 out]
          }
          frame "Btn_error" {
            # "// Get TSL error code"
            n166 = local read "TSL"() -> (w240:refnum<k24>)
            n167 = call "Get_System_Error.vi"("error in (no error)"=w238, ".NET Reference in"=w240) -> ("error"=→"txttsl_err":string)  [unwired: 7 in, 2 out]
          }
          frame "Btn_GetLD" {
            # "// Get LD Status"
            n168 = local read "TSL"() -> (w243:refnum<k24>)
            n169 = call "Get_LD_Status.vi"("error in (no error)"=w242, ".NET Reference in"=w243) -> ("status"=→"txtlds":enum16{"LD_OFF", "LD_ON", ""})  [unwired: 7 in, 2 out]
          }
          frame "BtnPower_mode" {
            # "// Get Power Mode"
            n170 = local read "TSL"() -> (w246:refnum<k24>)
            n171 = call "Get_Power_Mode.vi"("error in (no error)"=w244, ".NET Reference in"=w246) -> ("mode"=→"mode":enum16{"ACC", "APC", ""})  [unwired: 7 in, 2 out]
          }
          frame "BtnCoh_Status" {
            # "// Get coh Status"
            n172 = local read "TSL"() -> (w249:refnum<k24>)
            n173 = call "Get_Coh_Control_Status.vi"("error in (no error)"=w248, ".NET Reference in"=w249) -> ("status"=→"status":enum16{"Coh_OFF", "Coh_ON", ""})  [unwired: 7 in, 2 out]
          }
          frame "BtnShutter_Status" {
            # "// Get  shutter status"
            n174 = local read "TSL"() -> (w252:refnum<k24>)
            n175 = call "Get_Shutter_Status.vi"("error in (no error)"=w251, ".NET Reference in"=w252) -> ("status"=→"txtshutter":enum16{"Shutter_Open", "Shutter_Close", ""})  [unwired: 7 in, 2 out]
          }
          frame "BtnUnit" {
            # "// Get Unit"
            n176 = local read "TSL"() -> (w255:refnum<k24>)
            n177 = call "Get_Power_Unit.vi"("error in (no error)"=w254, ".NET Reference in"=w255) -> ("unit"=→"unit":enum16{"dBm", "mW", ""})  [unwired: 7 in, 2 out]
          }
          frame "BtnAtt_value" {
            # "// Get Att value"
            n178 = local read "TSL"() -> (w257:refnum<k24>)
            n179 = call "Get_Att_Value.vi"("error in (no error)"=w256, ".NET Reference in"=w257) -> ("att out"=→"txtreadatt":dbl)  [unwired: 7 in, 2 out]
          }
          frame "BtnPower_dBm" {
            # "// Get Setting power dBm"
            n180 = local read "TSL"() -> (w260:refnum<k24>)
            n181 = call "Get_Setting_Power_dBm.vi"("error in (no error)"=w259, ".NET Reference in"=w260) -> ("pow out"=→"txtreadpow":dbl)  [unwired: 7 in, 2 out]
          }
          frame "BtnPower_mW" {
            # "// Get Setting power mW"
            n182 = local read "TSL"() -> (w263:refnum<k24>)
            n183 = call "Get_Setting_Power_mW.vi"("error in (no error)"=w262, ".NET Reference in"=w263) -> ("pow out"=→"txtreadmw":dbl)  [unwired: 7 in, 2 out]
          }
          frame "Btnmonitor_dBm" {
            # "// Get Monitor power dBm"
            n184 = local read "TSL"() -> (w267:refnum<k24>)
            n185 = call "Get_Monitor_Power_dBm.vi"("error in (no error)"=w265, ".NET Reference in"=w267) -> ("power out"=→"txtreadmoni":dbl)  [unwired: 7 in, 2 out]
          }
          frame "Btnmonitor_mW" {
            (unwired) 0.0 ("pow")
            # "// Get Monitor power mW"
            n186 = local read "TSL"() -> (w270:refnum<k24>)
            n187 = call "Get_Monitor_Power_mW.vi"("error in (no error)"=w268, ".NET Reference in"=w270) -> ("pow out"=→"txtradmoni_mw":dbl)  [unwired: 7 in, 2 out]
          }
          frame "Btn_SetWavelength_Parameters" {
            # "// set Wavelength"
            n188 = local read "TSL"() -> (w279:refnum<k24>)
            n189 = call "Set_Sweep_Wavelength.vi"("error in (no error)"=w271, "Stop wavelength"="txtstop", "Start wavelength"="txtstart", ".NET Reference in"=w279) -> ("error out"=w272:errorcluster, ".NET Reference out"=w275:refnum<k24>)  [unwired: 6 in]
            n190 = call "Set_Wavelength_Step.vi"("error in (no error)"=w272, "wave step"="txtstep", ".NET Reference in"=w275) -> ("error out"=w273:errorcluster, ".NET Reference out"=w274:refnum<k24>)  [unwired: 7 in]
            n191 = call "Set_Trigger_Step.vi"("error in (no error)"=w273, "Trigger step"="txtstep", ".NET Reference in"=w274) -> ()  [unwired: 7 in, 2 out]
          }
          frame "Btn_Other" {
            # "// Set Sweep Parameters"
            n192 = local read "Target"() -> (w281:enum32{"rdo550", "rdo570", "rdo770"})
            n193 = case shown="\"rdo570\"" w281 {
              tunnel: ["txtspeed(550)" "Speed(570)"] -> w297
              frame "rdo550", Default {
              }
              frame "rdo570" {
              }
            }
            n194 = local read "TSL"() -> (w296:refnum<k24>)
            n195 = call "Set_Sweep_Speed.vi"("error in (no error)"=w280, "Speed(nm/sec)"=w297, ".NET Reference in"=w296) -> ("error out"=w284:errorcluster, ".NET Reference out"=w285:refnum<k24>)  [unwired: 7 in]
            n196 = call "Set_Sweep_Delay.vi"("error in (no error)"=w284, "Delay time(sec)"="txtdelay", ".NET Reference in"=w285) -> ("error out"=w286:errorcluster, ".NET Reference out"=w287:refnum<k24>)  [unwired: 7 in]
            n197 = call "Set_Sweep_Cycle.vi"("error in (no error)"=w286, "cycle"="txtcycle", ".NET Reference in"=w287) -> ("error out"=w288:errorcluster, ".NET Reference out"=w292:refnum<k24>)  [unwired: 7 in]
            n198 = call "Set_Sweep_Mode_Parameters.vi"("Start mode"="cmbtin", "Sweep Mode"="cmbsm", "error in (no error)"=w288, "Trigger input"="cmbst_mod", "Trigger output"="cmbtout", ".NET Reference in"=w292) -> ("error out"=w283:errorcluster, "Reference out"=w282:refnum<k24>)  [unwired: 4 in]
            n199 = case shown="\"rdo770\"" w281 {
              tunnel: w283 -> [_ w302 w305]
              tunnel: w282 -> [_ w301 w304]
              frame "rdo550", Default {
              }
              frame "rdo570" {
                n200 = call "Set_TriggerOutput_Source.vi"("error in (no error)"=w302, "mode"="cmbTrigger_Source", ".NET Reference in"=w301) -> ()  [unwired: 7 in, 2 out]
              }
              frame "rdo770" {
                n201 = local read "cmbTrigger_Source"() -> (w303:u16)
                n202 = call "Set_TriggerOutput_Source.vi"("error in (no error)"=w305, "mode"=w303, ".NET Reference in"=w304) -> ()  [unwired: 7 in, 2 out]
              }
            }
          }
          frame "BtnGet_setting" {
            # "// get sweep paremters"
            n203 = local read "TSL"() -> (w339:refnum<k24>)
            n204 = call "Get_Sweep_Mode.vi"("error in (no error)"=w307, ".NET Reference in"=w339) -> ("error out"=w336:errorcluster, "smod"=→"Sweep Mode":T3, ".NET Reference out"=w337:refnum<k24>)  [unwired: 7 in]
            n205 = call "Get_Input_Trigger_Mode.vi"("error in (no error)"=w336, ".NET Reference in"=w337) -> ("error out"=w312:errorcluster, "mode"=→"Trigger input":enum16{"Disable", "Enable", ""}, ".NET Reference out"=w311:refnum<k24>)  [unwired: 7 in]
            n206 = call "Get_Trigger_Output_Mode.vi"("error in (no error)"=w312, ".NET Reference in"=w311) -> ("error out"=w313:errorcluster, "mode"=→"Trigger output":enum16{"None", "Stop", "Start", "Step", ""}, ".NET Reference out"=w314:refnum<k24>)  [unwired: 7 in]
            n207 = call "Get_Sweep_Start_Mode.vi"("error in (no error)"=w313, ".NET Reference in"=w314) -> ("error out"=w316:errorcluster, "mode"=→"Start mode":enum16{"Normal", "WaitingforTrigger", ""}, ".NET Reference out"=w315:refnum<k24>)  [unwired: 7 in]
            n208 = call "Get_Sweep_Speed.vi"("error in (no error)"=w316, ".NET Reference in"=w315) -> ("error out"=w318:errorcluster, "speed out"=→"Speed(nm/sec)":dbl, ".NET Reference out"=w317:refnum<k24>)  [unwired: 7 in]
            n209 = call "Get_Sweep_Wavelength.vi"("error in (no error)"=w318, ".NET Reference in"=w317) -> ("error out"=w319:errorcluster, "endwave out"=→"Stop wavelength":dbl, "startwave out"=→"Start wavelength":dbl, ".NET Reference out"=w320:refnum<k24>)  [unwired: 6 in]
            n210 = call "Get_Sweep_Delay.vi"("error in (no error)"=w319, ".NET Reference in"=w320) -> ("error out"=w323:errorcluster, "delay out"=→"Delay time(sec)":dbl, ".NET Reference out"=w321:refnum<k24>)  [unwired: 7 in]
            n211 = call "Get_Sweep_Cycle.vi"("error in (no error)"=w323, ".NET Reference in"=w321) -> ("error out"=w324:errorcluster, "times out"=→"cycle":i32, ".NET Reference out"=w322:refnum<k24>)  [unwired: 7 in]
            n212 = call "Get_Wavelength_Step.vi"("error in (no error)"=w324, ".NET Reference in"=w322) -> ("error out"=w325:errorcluster, "wavestep out"=→"Wavelength step":dbl, ".NET Reference out"=w326:refnum<k24>)  [unwired: 7 in]
            n213 = local read "Target"() -> (w308:enum32{"rdo550", "rdo570", "rdo770"})
            n214 = call "Get_Trigger_Step.vi"("error in (no error)"=w325, ".NET Reference in"=w326) -> ("error out"=w310:errorcluster, "triggerstep"=→"Trigger step":dbl, "Reference out"=w309:refnum<k24>)  [unwired: 7 in]
            n215 = case shown="\"rdo770\"" w308 {
              tunnel: w310 -> [_ w342 w344]
              tunnel: w309 -> [_ w341 w345]
              frame "rdo550", Default {
              }
              frame "rdo570" {
                n216 = call "Get_TriggerOutput_Source.vi"("error in (no error)"=w342, ".NET Reference in"=w341) -> ("mode"=→"Trigger Source":enum16{"Wavelength", "Time", ""})  [unwired: 7 in, 2 out]
              }
              frame "rdo770" {
                n217 = call "Get_TriggerOutput_Source.vi"("error in (no error)"=w344, ".NET Reference in"=w345) -> ("mode"=w343:enum16{"Wavelength", "Time", ""})  [unwired: 7 in, 2 out]
                n218 = local write "Trigger Source"(w343) -> ()
              }
            }
          }
          frame "Btn_Waiting" {
            # "// Waititng for sweep status"
            n219 = flat-sequence {
              tunnel: [w354] -> w348
              tunnel: w346 -> [w355]
              tunnel: [w359] -> w347
              frame #0 {
                n220 = Tick Count (ms)() -> (millisecond timer value=w354:u32)
              }
              frame #1 {
                n221 = local read "TSL"() -> (w358:refnum<k24>)
                n222 = call "Waiting_Sweep_Status.vi"("error in (no error)"=w355, "status"="Status", "Wait time(msec)"="Wait time(msec)", ".NET Reference in"=w358) -> ()  [unwired: 6 in, 2 out]
              }
              frame #2 {
                n223 = Tick Count (ms)() -> (millisecond timer value=w359:u32)
              }
            }
            n224 = Subtract(x=w347, y=w348) -> (x-y=w349:u32)
            n225 = Number To Decimal String(number=w349) -> (decimal integer string=w352:string)  [unwired: 1 in]
            n226 = Concatenate Strings("waiting time:", w352, "msec") -> (w350:string)
            n227 = One Button Dialog(message=w350) -> ()  [unwired: 1 in, 1 out]
          }
          frame "Btn_Status" {
            # "// Get Sweep status"
            n228 = local read "TSL"() -> (w362:refnum<k24>)
            n229 = call "Get_Sweep_Status.vi"("error in (no error)"=w361, ".NET Reference in"=w362) -> ("status"=→"txtg_sweep_su":i32)  [unwired: 7 in, 2 out]
          }
          frame "Btn_GetLogg" {
            # "// Get Sweep Loggdata"
            n230 = local read "TSL"() -> (w365:refnum<k24>)
            n231 = call "Get_Logging_Data.vi"("error in (no error)"=w364, ".NET Reference in"=w365) -> ("data out"=w363:dbl[])  [unwired: 6 in, 3 out]
            n232 = call-poly <vilib>:"Write To Spreadsheet File.vi"("transpose? (no:F)"=TRUE, "1D data"=w363) -> ()  [unwired: 6 in, 1 out]
          }
          frame "Btn_Current" {
            # "// Get current cycles"
            n233 = local read "TSL"() -> (w369:refnum<k24>)
            n234 = call "Get_Sweep_Count.vi"("error in (no error)"=w367, ".NET Reference in"=w369) -> ("count out"=→"txtcurrentc":i32)  [unwired: 7 in, 2 out]
          }
          frame "Btn_Minstep" {
            # "Calucrate Minimum trigger step from sweep speed"
            n235 = local read "TSL"() -> (w371:refnum<k24>)
            n236 = call "Cal_MinimumTriggerStep_from_SweepSpeed.vi"("error in (no error)"=w370, "speed"="txtspeed", ".NET Reference in"=w371) -> ("triggerstep out"=w372:dbl)  [unwired: 6 in, 2 out]
            n237 = Number To Fractional String(number=w372) -> (F-format string=w374:string)  [unwired: 3 in]
            n238 = Concatenate Strings("Minimum trigger step = ", w374, "nm") -> (w375:string)
            n239 = One Button Dialog(message=w375) -> ()  [unwired: 1 in, 1 out]
          }
          frame "Btn_Start" {
            # "// Sweep Start"
            n240 = local read "TSL"() -> (w379:refnum<k24>)
            n241 = call "Sweep_Start.vi"("error in (no error)"=w378, ".NET Reference in"=w379) -> ()  [unwired: 8 in, 2 out]
          }
          frame "Btn_Pause" {
            # "// Sweep Pause"
            n242 = local read "TSL"() -> (w381:refnum<k24>)
            n243 = call "Sweep_Pause.vi"("error in (no error)"=w380, ".NET Reference in"=w381) -> ()  [unwired: 8 in, 2 out]
          }
          frame "Btn_ReStart" {
            # "// Sweep Restart"
            n244 = local read "TSL"() -> (w383:refnum<k24>)
            n245 = call "Sweep_Restart.vi"("error in (no error)"=w382, ".NET Reference in"=w383) -> ()  [unwired: 8 in, 2 out]
          }
          frame "Btn_Stop" {
            # "// Sweep Stop"
            n246 = local read "TSL"() -> (w385:refnum<k24>)
            n247 = call "Sweep_Pause.vi"("error in (no error)"=w384, ".NET Reference in"=w385) -> ("error out"=w386:errorcluster, "Reference out"=w387:refnum<k24>)  [unwired: 8 in]
            n248 = call "Sweep_Stop.vi"("error in (no error)"=w386, ".NET Reference in"=w387) -> ()  [unwired: 8 in, 2 out]
          }
          frame "Btn_SoftwareTrigger" {
            # "// software trigger"
            n249 = local read "TSL"() -> (w389:refnum<k24>)
            n250 = call "Set_Software_Trigger.vi"("error in (no error)"=w388, ".NET Reference in"=w389) -> ()  [unwired: 8 in, 2 out]
          }
          frame "Get IP Address" {
            n251 = local read "TSL"() -> (w392:refnum<k24>)
            n252 = call "Get_IPAddress.vi"("error in (no error)"=w390, ".NET Reference in"=w392) -> ("address"=→"IP Address":string)  [unwired: 7 in, 2 out]
          }
          frame "Get LAN Port" {
            n253 = local read "TSL"() -> (w395:refnum<k24>)
            n254 = call "Get_LAN_Portnumber.vi"("error in (no error)"=w393, ".NET Reference in"=w395) -> ("portnum"=→"LAN Port number":i32)  [unwired: 7 in, 2 out]
          }
          frame "Communication" {
            n255 = local read "Communication"() -> (w396:T2)
            n256 = case shown="\"rdiNI488\", Default" w396 {
              frame "rdiNI488", Default {
                w397 = T6."Enabled" ("禁用")
                n257 = property on="rdiCrLf" class="Bool (strict)"("DisabledEnum"=w397) -> ()  [unwired: 2 in, 2 out]
                n258 = property on="rdiLf" class="Bool (strict)"("DisabledEnum"=w397) -> ()  [unwired: 2 in, 2 out]
              }
              frame "rdiLAN" {
                w398 = T6."Disabled and Grayed Out" ("禁用")
                n259 = local write "Port number"(5000.0 ("Port number")) -> ()
                n260 = property on="rdiCr" class="Bool (strict)"("Key Focus"=TRUE ("键选中")) -> ()  [unwired: 2 in, 2 out]
                n261 = property on="rdiLf" class="Bool (strict)"("DisabledEnum"=w398) -> ()  [unwired: 2 in, 2 out]
                n262 = property on="rdiCrLf" class="Bool (strict)"("DisabledEnum"=w398) -> ()  [unwired: 2 in, 2 out]
              }
              frame "rdiUSB" {
                w401 = T6."Disabled and Grayed Out" ("禁用")
                n263 = local read "USB device number"() -> (w403:string)
                n264 = local write "Port number"(5000.0 ("Port number")) -> ()
                n265 = local write "Address/Device number"(w403) -> ()
                n266 = property on="rdiCr" class="Bool (strict)"("Key Focus"=TRUE ("键选中")) -> ()  [unwired: 2 in, 2 out]
                n267 = property on="rdiCrLf" class="Bool (strict)"("DisabledEnum"=w401) -> ()  [unwired: 2 in, 2 out]
                n268 = property on="rdiLf" class="Bool (strict)"("DisabledEnum"=w401) -> ()  [unwired: 2 in, 2 out]
              }
            }
          }
        }
      }
      frame Error {
      }
    }
  }
  n269 = while {
    tunnel: w1 -> [w411]
    shift-right: [w407] -> w5
    shift-left: w6 -> [w406]
    stop <- w408 stop-if-true
    n270 = event shown="[41] \"Btn_Other\": Value Change" {
      selector: _ -> [_ _ _ _ _ _ _ _ _ _ _ _ _ _ _ _ _ _ _ _ _ _ _ _ _ _ _ _ _ _ _ _ _ _ _ _ _ _ _ _ _ _ _ _ _ _ _ _ _ _ _ _ _ _ _ _ _]
      dyn-events: _ -> [_ _ _ _ _ _ _ _ _ _ _ _ _ _ _ _ _ _ _ _ _ _ _ _ _ _ _ _ _ _ _ _ _ _ _ _ _ _ _ _ _ _ _ _ _ _ _ _ _ _ _ _ _ _ _ _ _]
      timeout: _ -> [_ _ _ _ _ _ _ _ _ _ _ _ _ _ _ _ _ _ _ _ _ _ _ _ _ _ _ _ _ _ _ _ _ _ _ _ _ _ _ _ _ _ _ _ _ _ _ _ _ _ _ _ _ _ _ _ _]
      tunnel: w411 -> [w416 w421 w425 w428 w433 w438 w442 w444 w449 w452 w456 w460 w464 w468 w472 w476 w480 w484 w488 w492 w496 w500 w504 w508 w512 w516 w520 w524 w528 w532 w536 w540 w544 w548 w552 w556 w560 w564 w568 w572 w576 w580 w584 w588 w592 w596 w600 w604 w608 w612 w616 _ w621 w625 w629 w633 w637]
      tunnel: w406 -> [w415 w420 w424 w427 w432 w437 w441 w443 w448 w453 w457 w459 w463 w467 w471 w475 w479 w483 w487 w491 w495 w499 w503 w507 w511 w515 w519 w523 w527 w531 w535 w539 w543 w547 w551 w555 w559 w563 w567 w571 w575 w579 w583 w587 w591 w595 w599 w603 w607 w611 w615 _ w620 w624 w628 w632 w636]
      tunnel: [w414 w419 w422 w426 w430 w435 w439 w445 w447 w451 w455 w461 w465 w469 w473 w477 w481 w485 w489 w493 w497 w501 w505 w509 w513 w517 w521 w525 w529 w533 w537 w541 w545 w549 w553 w557 w561 w565 w569 w573 w577 w581 w585 w589 w593 w597 w601 w605 w609 w613 w617 _ w622 w626 w630 w634 w638] -> w407
      tunnel: [FALSE ("stop") FALSE ("stop") _ _ w431 _ _ _ _ _ _ _ _ _ _ _ _ _ _ _ _ _ _ _ _ _ _ _ _ _ _ _ _ _ _ _ _ _ _ _ _ _ _ _ _ _ _ _ _ _ _ TRUE ("timed out?") _ _ _ _ _] -> w409
      event "Btn_Connect": Value Change {
        n271 = event-data() -> ()  [unwired: 1 in, 1 out]
        n272 = Enqueue Element(queue=w416, element="Btn_Connect" ("元素"), error in (no error)=w415) -> (error out=w414:errorcluster)  [unwired: 1 in, 2 out]
      }
      event "btnSplit": Value Change {
        n273 = event-data() -> ()  [unwired: 1 in, 1 out]
        n274 = Enqueue Element(queue=w421, element="btnSplit" ("元素"), error in (no error)=w420) -> (error out=w419:errorcluster)  [unwired: 1 in, 2 out]
      }
      event "btnGet_Visa": Value Change {
        n275 = event-data() -> ()  [unwired: 1 in, 1 out]
        n276 = Enqueue Element(queue=w425, element="btnGet_Visa" ("元素"), error in (no error)=w424) -> (error out=w422:errorcluster)  [unwired: 1 in, 2 out]
      }
      event "btnUsb_resouce": Value Change {
        n277 = event-data() -> ()  [unwired: 1 in, 1 out]
        n278 = Enqueue Element(queue=w428, element="btnUsb_resouce" ("元素"), error in (no error)=w427) -> (error out=w426:errorcluster)  [unwired: 1 in, 2 out]
      }
      event "Usb resouce": Value Change {
        n279 = event-data() -> ()  [unwired: 1 in, 1 out]
        n280 = Enqueue Element(queue=w433, element="Usbresouce_Select" ("元素"), error in (no error)=w432) -> (timed out?=w431:bool, error out=w430:errorcluster)  [unwired: 1 in, 1 out]
      }
      event "Get IP Address": Value Change {
        n281 = event-data() -> ()  [unwired: 1 in, 1 out]
        n282 = Enqueue Element(queue=w438, element="Get IP Address" ("元素"), error in (no error)=w437) -> (error out=w435:errorcluster)  [unwired: 1 in, 2 out]
      }
      event "Get LAN Port": Value Change {
        n283 = event-data() -> ()  [unwired: 1 in, 1 out]
        n284 = Enqueue Element(queue=w442, element="Get LAN Port" ("元素"), error in (no error)=w441) -> (error out=w439:errorcluster)  [unwired: 1 in, 2 out]
      }
      event "Btn_DisConnect": Value Change {
        n285 = event-data() -> ()  [unwired: 1 in, 1 out]
        n286 = Enqueue Element(queue=w444, element="Btn_DisConnect" ("元素"), error in (no error)=w443) -> (error out=w445:errorcluster)  [unwired: 1 in, 2 out]
      }
      event "BtnLD_ON": Value Change {
        n287 = event-data() -> ()  [unwired: 1 in, 1 out]
        n288 = Enqueue Element(queue=w449, element="BtnLD_ON" ("元素"), error in (no error)=w448) -> (error out=w447:errorcluster)  [unwired: 1 in, 2 out]
      }
      event "BtnLD_OFF": Value Change {
        n289 = event-data() -> ()  [unwired: 1 in, 1 out]
        n290 = Enqueue Element(queue=w452, element="BtnLD_OFF" ("元素"), error in (no error)=w453) -> (error out=w451:errorcluster)  [unwired: 1 in, 2 out]
      }
      event "BtnCoh_ON": Value Change {
        n291 = event-data() -> ()  [unwired: 1 in, 1 out]
        n292 = Enqueue Element(queue=w456, element="BtnCoh_ON" ("元素"), error in (no error)=w457) -> (error out=w455:errorcluster)  [unwired: 1 in, 2 out]
      }
      event "BtnCoh_OFF": Value Change {
        n293 = event-data() -> ()  [unwired: 1 in, 1 out]
        n294 = Enqueue Element(queue=w460, element="BtnCoh_OFF" ("元素"), error in (no error)=w459) -> (error out=w461:errorcluster)  [unwired: 1 in, 2 out]
      }
      event "BtnShutter_Open": Value Change {
        n295 = event-data() -> ()  [unwired: 1 in, 1 out]
        n296 = Enqueue Element(queue=w464, element="BtnShutter_Open" ("元素"), error in (no error)=w463) -> (error out=w465:errorcluster)  [unwired: 1 in, 2 out]
      }
      event "BtnShutter_Close": Value Change {
        n297 = event-data() -> ()  [unwired: 1 in, 1 out]
        n298 = Enqueue Element(queue=w468, element="BtnShutter_Close" ("元素"), error in (no error)=w467) -> (error out=w469:errorcluster)  [unwired: 1 in, 2 out]
      }
      event "BtnAPC": Value Change {
        n299 = event-data() -> ()  [unwired: 1 in, 1 out]
        n300 = Enqueue Element(queue=w472, element="BtnAPC" ("元素"), error in (no error)=w471) -> (error out=w473:errorcluster)  [unwired: 1 in, 2 out]
      }
      event "BtnACC": Value Change {
        n301 = event-data() -> ()  [unwired: 1 in, 1 out]
        n302 = Enqueue Element(queue=w476, element="BtnACC" ("元素"), error in (no error)=w475) -> (error out=w477:errorcluster)  [unwired: 1 in, 2 out]
      }
      event "BtndBm": Value Change {
        n303 = event-data() -> ()  [unwired: 1 in, 1 out]
        n304 = Enqueue Element(queue=w480, element="BtndBm" ("元素"), error in (no error)=w479) -> (error out=w481:errorcluster)  [unwired: 1 in, 2 out]
      }
      event "BtnmW": Value Change {
        n305 = event-data() -> ()  [unwired: 1 in, 1 out]
        n306 = Enqueue Element(queue=w484, element="BtnmW" ("元素"), error in (no error)=w483) -> (error out=w485:errorcluster)  [unwired: 1 in, 2 out]
      }
      event "Btn_SetATT": Value Change {
        n307 = event-data() -> ()  [unwired: 1 in, 1 out]
        n308 = Enqueue Element(queue=w488, element="Btn_SetATT" ("元素"), error in (no error)=w487) -> (error out=w489:errorcluster)  [unwired: 1 in, 2 out]
      }
      event "Btn_SetdBm": Value Change {
        n309 = event-data() -> ()  [unwired: 1 in, 1 out]
        n310 = Enqueue Element(queue=w492, element="Btn_SetdBm" ("元素"), error in (no error)=w491) -> (error out=w493:errorcluster)  [unwired: 1 in, 2 out]
      }
      event "Btn_SetmW": Value Change {
        n311 = event-data() -> ()  [unwired: 1 in, 1 out]
        n312 = Enqueue Element(queue=w496, element="Btn_SetmW" ("元素"), error in (no error)=w495) -> (error out=w497:errorcluster)  [unwired: 1 in, 2 out]
      }
      event "Btn_SetWavelength": Value Change {
        n313 = event-data() -> ()  [unwired: 1 in, 1 out]
        n314 = Enqueue Element(queue=w500, element="Btn_SetWavelength" ("元素"), error in (no error)=w499) -> (error out=w501:errorcluster)  [unwired: 1 in, 2 out]
      }
      event "Btn_SetFrequency": Value Change {
        n315 = event-data() -> ()  [unwired: 1 in, 1 out]
        n316 = Enqueue Element(queue=w504, element="Btn_SetFrequency" ("元素"), error in (no error)=w503) -> (error out=w505:errorcluster)  [unwired: 1 in, 2 out]
      }
      event "Btn_SetFinetuning": Value Change {
        n317 = event-data() -> ()  [unwired: 1 in, 1 out]
        n318 = Enqueue Element(queue=w508, element="Btn_SetFinetuning" ("元素"), error in (no error)=w507) -> (error out=w509:errorcluster)  [unwired: 1 in, 2 out]
      }
      event "Btn_Wavelength": Value Change {
        n319 = event-data() -> ()  [unwired: 1 in, 1 out]
        n320 = Enqueue Element(queue=w512, element="Btn_Wavelength" ("元素"), error in (no error)=w511) -> (error out=w513:errorcluster)  [unwired: 1 in, 2 out]
      }
      event "Btn_Frequency": Value Change {
        n321 = event-data() -> ()  [unwired: 1 in, 1 out]
        n322 = Enqueue Element(queue=w516, element="Btn_Frequency" ("元素"), error in (no error)=w515) -> (error out=w517:errorcluster)  [unwired: 1 in, 2 out]
      }
      event "Btn_Fine": Value Change {
        n323 = event-data() -> ()  [unwired: 1 in, 1 out]
        n324 = Enqueue Element(queue=w520, element="Btn_Fine" ("元素"), error in (no error)=w519) -> (error out=w521:errorcluster)  [unwired: 1 in, 2 out]
      }
      event "Btn_Busy": Value Change {
        n325 = event-data() -> ()  [unwired: 1 in, 1 out]
        n326 = Enqueue Element(queue=w524, element="Btn_Busy" ("元素"), error in (no error)=w523) -> (error out=w525:errorcluster)  [unwired: 1 in, 2 out]
      }
      event "Btn_Stangby": Value Change {
        n327 = event-data() -> ()  [unwired: 1 in, 1 out]
        n328 = Enqueue Element(queue=w528, element="Btn_Stangby" ("元素"), error in (no error)=w527) -> (error out=w529:errorcluster)  [unwired: 1 in, 2 out]
      }
      event "Btn_error": Value Change {
        n329 = event-data() -> ()  [unwired: 1 in, 1 out]
        n330 = Enqueue Element(queue=w532, element="Btn_error" ("元素"), error in (no error)=w531) -> (error out=w533:errorcluster)  [unwired: 1 in, 2 out]
      }
      event "Btn_GetLD": Value Change {
        n331 = event-data() -> ()  [unwired: 1 in, 1 out]
        n332 = Enqueue Element(queue=w536, element="Btn_GetLD" ("元素"), error in (no error)=w535) -> (error out=w537:errorcluster)  [unwired: 1 in, 2 out]
      }
      event "BtnPower_mode": Value Change {
        n333 = event-data() -> ()  [unwired: 1 in, 1 out]
        n334 = Enqueue Element(queue=w540, element="BtnPower_mode" ("元素"), error in (no error)=w539) -> (error out=w541:errorcluster)  [unwired: 1 in, 2 out]
      }
      event "BtnCoh_Status": Value Change {
        n335 = event-data() -> ()  [unwired: 1 in, 1 out]
        n336 = Enqueue Element(queue=w544, element="BtnCoh_Status" ("元素"), error in (no error)=w543) -> (error out=w545:errorcluster)  [unwired: 1 in, 2 out]
      }
      event "BtnShutter_Status": Value Change {
        n337 = event-data() -> ()  [unwired: 1 in, 1 out]
        n338 = Enqueue Element(queue=w548, element="BtnShutter_Status" ("元素"), error in (no error)=w547) -> (error out=w549:errorcluster)  [unwired: 1 in, 2 out]
      }
      event "BtnUnit": Value Change {
        n339 = event-data() -> ()  [unwired: 1 in, 1 out]
        n340 = Enqueue Element(queue=w552, element="BtnUnit" ("元素"), error in (no error)=w551) -> (error out=w553:errorcluster)  [unwired: 1 in, 2 out]
      }
      event "BtnAtt_value": Value Change {
        n341 = event-data() -> ()  [unwired: 1 in, 1 out]
        n342 = Enqueue Element(queue=w556, element="BtnAtt_value" ("元素"), error in (no error)=w555) -> (error out=w557:errorcluster)  [unwired: 1 in, 2 out]
      }
      event "BtnPower_dBm": Value Change {
        n343 = event-data() -> ()  [unwired: 1 in, 1 out]
        n344 = Enqueue Element(queue=w560, element="BtnPower_dBm" ("元素"), error in (no error)=w559) -> (error out=w561:errorcluster)  [unwired: 1 in, 2 out]
      }
      event "BtnPower_mW": Value Change {
        n345 = event-data() -> ()  [unwired: 1 in, 1 out]
        n346 = Enqueue Element(queue=w564, element="BtnPower_mW" ("元素"), error in (no error)=w563) -> (error out=w565:errorcluster)  [unwired: 1 in, 2 out]
      }
      event "Btnmonitor_dBm": Value Change {
        n347 = event-data() -> ()  [unwired: 1 in, 1 out]
        n348 = Enqueue Element(queue=w568, element="Btnmonitor_dBm" ("元素"), error in (no error)=w567) -> (error out=w569:errorcluster)  [unwired: 1 in, 2 out]
      }
      event "Btnmonitor_mW": Value Change {
        n349 = event-data() -> ()  [unwired: 1 in, 1 out]
        n350 = Enqueue Element(queue=w572, element="Btnmonitor_mW" ("元素"), error in (no error)=w571) -> (error out=w573:errorcluster)  [unwired: 1 in, 2 out]
      }
      event "Btn_SetWavelength_Parameters": Value Change {
        n351 = event-data() -> ()  [unwired: 1 in, 1 out]
        n352 = Enqueue Element(queue=w576, element="Btn_SetWavelength_Parameters" ("元素"), error in (no error)=w575) -> (error out=w577:errorcluster)  [unwired: 1 in, 2 out]
      }
      event "Btn_Other": Value Change {
        n353 = event-data() -> ()  [unwired: 1 in, 1 out]
        n354 = Enqueue Element(queue=w580, element="Btn_Other" ("元素"), error in (no error)=w579) -> (error out=w581:errorcluster)  [unwired: 1 in, 2 out]
      }
      event "BtnGet_setting": Value Change {
        n355 = event-data() -> ()  [unwired: 1 in, 1 out]
        n356 = Enqueue Element(queue=w584, element="BtnGet_setting" ("元素"), error in (no error)=w583) -> (error out=w585:errorcluster)  [unwired: 1 in, 2 out]
      }
      event "Btn_Waiting": Value Change {
        n357 = event-data() -> ()  [unwired: 1 in, 1 out]
        n358 = Enqueue Element(queue=w588, element="Btn_Waiting" ("元素"), error in (no error)=w587) -> (error out=w589:errorcluster)  [unwired: 1 in, 2 out]
      }
      event "Get speed table": Value Change {
        n359 = event-data() -> ()  [unwired: 1 in, 1 out]
        n360 = Enqueue Element(queue=w592, element="Get speed table" ("元素"), error in (no error)=w591) -> (error out=w593:errorcluster)  [unwired: 1 in, 2 out]
      }
      event "Target": Value Change {
        n361 = event-data() -> ()  [unwired: 1 in, 1 out]
        n362 = Enqueue Element(queue=w596, element="Target" ("元素"), error in (no error)=w595) -> (error out=w597:errorcluster)  [unwired: 1 in, 2 out]
      }
      event "Communication": Value Change {
        n363 = event-data() -> ()  [unwired: 1 in, 1 out]
        n364 = Enqueue Element(queue=w600, element="Communication" ("元素"), error in (no error)=w599) -> (error out=w601:errorcluster)  [unwired: 1 in, 2 out]
      }
      event "Btn_Status": Value Change {
        n365 = event-data() -> ()  [unwired: 1 in, 1 out]
        n366 = Enqueue Element(queue=w604, element="Btn_Status" ("元素"), error in (no error)=w603) -> (error out=w605:errorcluster)  [unwired: 1 in, 2 out]
      }
      event "Btn_GetLogg": Value Change {
        n367 = event-data() -> ()  [unwired: 1 in, 1 out]
        n368 = Enqueue Element(queue=w608, element="Btn_GetLogg" ("元素"), error in (no error)=w607) -> (error out=w609:errorcluster)  [unwired: 1 in, 2 out]
      }
      event "Btn_Current": Value Change {
        n369 = event-data() -> ()  [unwired: 1 in, 1 out]
        n370 = Enqueue Element(queue=w612, element="Btn_Current" ("元素"), error in (no error)=w611) -> (error out=w613:errorcluster)  [unwired: 1 in, 2 out]
      }
      event "Btn_Minstep": Value Change {
        n371 = event-data() -> ()  [unwired: 1 in, 1 out]
        n372 = Enqueue Element(queue=w616, element="Btn_Minstep" ("元素"), error in (no error)=w615) -> (error out=w617:errorcluster)  [unwired: 1 in, 2 out]
      }
      event Panel Close {
        n373 = event-data() -> ()  [unwired: 1 in, 1 out]
      }
      event "Btn_Start": Value Change {
        n374 = event-data() -> ()  [unwired: 1 in, 1 out]
        n375 = Enqueue Element(queue=w621, element="Btn_Start" ("元素"), error in (no error)=w620) -> (error out=w622:errorcluster)  [unwired: 1 in, 2 out]
      }
      event "Btn_Pause": Value Change {
        n376 = event-data() -> ()  [unwired: 1 in, 1 out]
        n377 = Enqueue Element(queue=w625, element="Btn_Pause" ("元素"), error in (no error)=w624) -> (error out=w626:errorcluster)  [unwired: 1 in, 2 out]
      }
      event "Btn_ReStart": Value Change {
        n378 = event-data() -> ()  [unwired: 1 in, 1 out]
        n379 = Enqueue Element(queue=w629, element="Btn_ReStart" ("元素"), error in (no error)=w628) -> (error out=w630:errorcluster)  [unwired: 1 in, 2 out]
      }
      event "Btn_Stop": Value Change {
        n380 = event-data() -> ()  [unwired: 1 in, 1 out]
        n381 = Enqueue Element(queue=w633, element="Btn_Stop" ("元素"), error in (no error)=w632) -> (error out=w634:errorcluster)  [unwired: 1 in, 2 out]
      }
      event "Btn_SoftwareTrigger": Value Change {
        n382 = event-data() -> ()  [unwired: 1 in, 1 out]
        n383 = Enqueue Element(queue=w637, element="Btn_SoftwareTrigger" ("元素"), error in (no error)=w636) -> (error out=w638:errorcluster)  [unwired: 1 in, 2 out]
      }
    }
    n384 = Unbundle By Name(w407) -> ("status"=w410:bool)
    n385 = Or(x=w410, y=w409) -> (x .or. y?=w408:bool)
  }
  n386 = Release Queue(queue=w1, error in (no error)=w5) -> ()  [unwired: 1 in, 3 out]
